vi "CRYWaveform Resampling.vi"(10 "New Sampling Rate":dbl, 11 "Wave":T1={"Waveform"={"X0"=0.0, "dX"=0.0, "Y"=[]}, "X data"=1, "Y data"=1, "Y axis"=1, "X unit"="s", "Y unit"="V", "Y dB ref"=1.0, "display Y"=TRUE, "display X"=TRUE, "Overload?"=FALSE, "Test Info"="", "Step No."=0, "Name"="", "protected"=FALSE, "Sqc history"=[], "Signal Channel ID"=0, "Plot Settings"={"Color"=0, "Interpolation"=0, "Point Style"=0, "Line Style"=0, "Point Color"=0, "Line Width"=0, "Bar Plot Style"=0, "Fill To"=0}, "AutoProtect"=FALSE} {"Y dB ref" format="%.1f"; "Y axis" items=["Log", "Lin"]; "Y data" items=["dB", "Lin"]; "X data" items=["dB", "Lin"]}) -> (3 "New Wave":T1={"Waveform"={"X0"=0.0, "dX"=0.0, "Y"=[]}, "X data"=1, "Y data"=1, "Y axis"=1, "X unit"="s", "Y unit"="V", "Y dB ref"=1.0, "display Y"=TRUE, "display X"=TRUE, "Overload?"=FALSE, "Test Info"="", "Step No."=0, "Name"="", "protected"=FALSE, "Sqc history"=[], "Signal Channel ID"=0, "Plot Settings"={"Color"=0, "Interpolation"=0, "Point Style"=0, "Line Style"=0, "Point Color"=0, "Line Width"=0, "Bar Plot Style"=0, "Fill To"=0}, "AutoProtect"=FALSE} {"Y dB ref" format="%.1f"; "Y axis" items=["Log", "Lin"]; "Y data" items=["dB", "Lin"]; "X data" items=["dB", "Lin"]})   [LabVIEW 2013]
uses:
  Typedef Control/CRYWaveform Cluster.ctl
  <vilib>/Analysis/2dsp.llb/Resample (constant to constant,single -channel).vi
  <vilib>/Analysis/NI_AALPro.lvlib
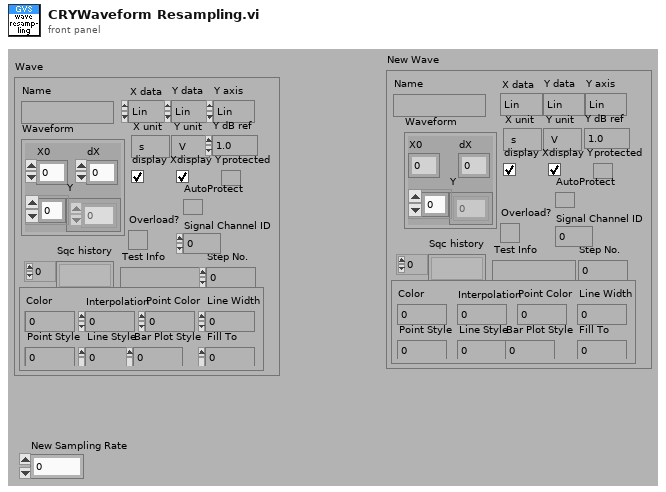
[diagram p1: front panel]
types:
  T1 = typedef "CRYWaveform Cluster.ctl" = cluster{"Waveform":cluster{"X0":dbl, "dX":dbl, "Y":sgl[]}, "X data":u16, "Y data":u16, "Y axis":u16, "X unit":string, "Y unit":string, "Y dB ref":dbl, "display Y":bool, "display X":bool, "Overload?":bool, "Test Info":string, "Step No.":i32, "Name":string, "protected":bool, "Sqc history":string[], "Signal Channel ID":i32, "Plot Settings":cluster{"Color":u32, "Interpolation":u8, "Point Style":u8, "Line Style":u8, "Point Color":u32, "Line Width":u8, "Bar Plot Style":u8, "Fill To":i16}, "AutoProtect":bool}
  T2 = cluster{"alias rejection (dB)":dbl, "normalized bandwidth":dbl}
  T3 = typedef "CRYStimulus Test Infor Cluster.ctl" = cluster{"Stimulus Type":string, "Signal Type":string, "In/Out":bool, "FAPS":cluster{"freq":dbl, "ampl":dbl, "cycles":dbl, "samples":i32}[], "Sampling Rate":dbl, "Samples":i32, "Analysis Param":string, "Resolution":u16, "Steps":u32, "Analysis Value":dbl[], "Diff Freq":dbl, "FStart":dbl, "FStop":dbl, "Calibration Param":string, "Anti Alias":dbl, "Level Out1":dbl, "Level Out2":dbl, "EQ":bool}
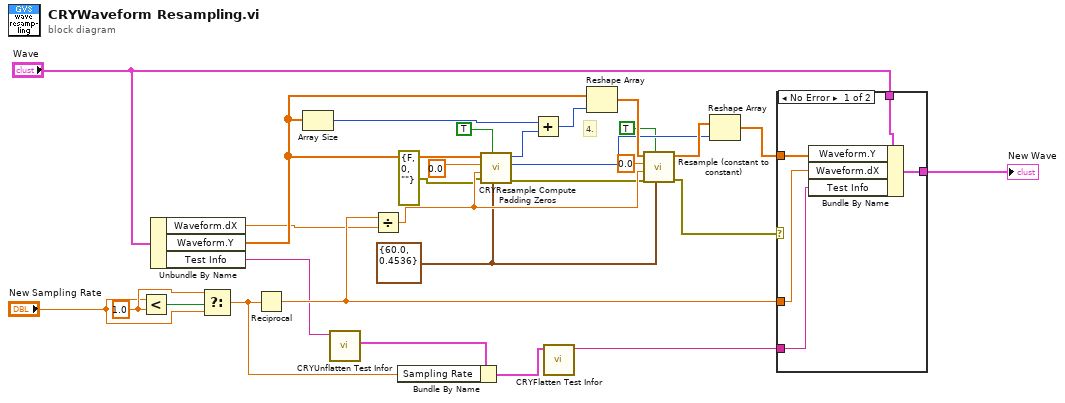
[diagram p0: block diagram]
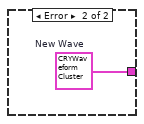
[diagram p2: hidden frame]
diagram:
  w19 = 1.0 ("y")
  w24 = T2 {"alias rejection (dB)"=60.0, "normalized bandwidth"=0.4536} ("FIR filter specifications")
  # "4."
  n1 = Less?(x="New Sampling Rate", y=w19) -> (x < y?=w20:bool)
  n2 = Unbundle By Name("Wave") -> ("Waveform.dX"=w11:dbl, "Waveform.Y"=w14:sgl[], "Test Info"=w5:string)
  n3 = Select(t=w19, s=w20, f="New Sampling Rate") -> (s? t:f=w3:dbl)
  n4 = Reciprocal(x=w3) -> (1/x=w13:dbl)
  n5 = Array Size(array=w14) -> (size(s)=w12:i32)
  n6 = call "CRYUnflatten Test Infor.vi"("Falattend test infor"=w5) -> ("unflattened test infor data"=w4:T3)  [unwired: 8 in, 1 out]
  n7 = Divide(x=w13, y=w11) -> (x/y=w26:dbl)
  n8 = Bundle By Name(cluster=w4, "Sampling Rate"=w3) -> (w2:T3)
  n9 = call "CRYResample Compute Padding Zeros.vi"("FIR filter specifications"=w24, "reset?"=TRUE, "error in (no error)"=errorcluster {"status"=FALSE, "code"=0, "source"=""}, "dt"=w26, "delay"=0.0, "X"=w14) -> ("error out"=w21:errorcluster, "length of Y"=w8:i32, "length of padding zeros"=w29:i32)  [unwired: 3 in]
  n10 = Add(x=w12, y=w29) -> (x+y=w28:i32)
  n11 = call "CRYFlatten Test Infor.vi"("Test Infor data"=w2) -> ("Fattened Data"=w1:string)  [unwired: 10 in]
  n12 = Reshape Array(w14, w28) -> (w25:sgl[])
  n13 = call-poly <vilib>:"Resample (constant to constant).vi"("FIR filter specifications"=w24, "reset?"=TRUE, "error in (no error)"=w21, "dt"=w26, "delay"=0.0, "X"=w25) -> ("error out"=w17:errorcluster, "Y"=w10:dbl[])  [unwired: 3 in, 1 out]
  n14 = Reshape Array(w10, w8) -> (w9:dbl[])
  n15 = case shown="No Error" w17 {
    tunnel: w13 -> [w32 _]
    tunnel: w9 -> [w33 _]
    tunnel: "Wave" -> [w34 _]
    tunnel: [w31 w35] -> w15
    tunnel: w1 -> [w30 _]
    frame No Error {
      n16 = Bundle By Name(cluster=w34, "Waveform.Y"=w33, "Waveform.dX"=w32, "Test Info"=w30) -> (w31:T1)
    }
    frame Error {
      w35 = T1 {"Waveform"={"X0"=0.0, "dX"=0.0, "Y"=[]}, "X data"=1, "Y data"=1, "Y axis"=1, "X unit"="s", "Y unit"="V", "Y dB ref"=1.0, "display Y"=TRUE, "display X"=TRUE, "Overload?"=FALSE, "Test Info"="", "Step No."=0, "Name"="", "protected"=FALSE, "Sqc history"=[], "Signal Channel ID"=0, "Plot Settings"={"Color"=0, "Interpolation"=0, "Point Style"=0, "Line Style"=0, "Point Color"=0, "Line Width"=0, "Bar Plot Style"=0, "Fill To"=0}, "AutoProtect"=FALSE}  # New Wave
    }
  }
  "New Wave" <- w15
